vi "RT Game POX.vi"() -> ()   [LabVIEW 2026]
uses:
  RT State.ctl
  SideSelector.ctl
  <extravilib>/ChannelInstances/Tag-bool/Read With Abort.vi
  <extravilib>/ChannelInstances/Tag-bool/Write With Abort.vi
  <vilib>/FPGAPlugInAG/cRIO-9047/niLvFpga_Open_cRIO-9047.vi
  <extravilib>/ChannelInstances/Tag-bool/Instantiate.vi
  <extravilib>/ChannelInstances/Tag-bool/EndpointRead.vi
  <vilib>/Utility/error.llb/Error Cluster From Error Code.vi
  <vilib>/rvi/errors/niLvFpgaAdjustHostInterfaceError.vi
  <extravilib>/ChannelInstances/Tag-bool/Endpoint.vi
  <vilib>/rvi/interface/nirviOpenFPGA/nirviOpenFPGA.xnode
  FPGA Bitfiles/speedofvight_FPGATarget_SpeedofVIightFPG_0-Md8D0SXKo.lvbitx
  VSandbox/Speed of VIight FPGA_v2.vi
  <vilib>/rvi/interface/nirviReadWriteControl/nirviReadWriteControl.xnode
  NiFpgaLv.dll
  <extravilib>/ChannelInstances/Tag-bool.lvlib
panel:
  in  "Effect":T1(ring)
  in  "Complete Game":bool
  in  "Abort Game":bool
  out "Player 2 Score Live":u32
  out "Player 1 Score Live":u32
  out "Player 2 Score":u32
  out "Player 1 Score":u32
  out "Enum":T2=enum."Game<>Conclude"
  in  "Game Length (s)":u32=2
  in  "Bonus Threshold":u64=30000
  in  "Commit to Game":bool
  in  "Stop Idle":bool
  out "Closing Loop":i32
  out "Main Loop":i32
  out "Idle Loop":i32
  in  "stop":bool
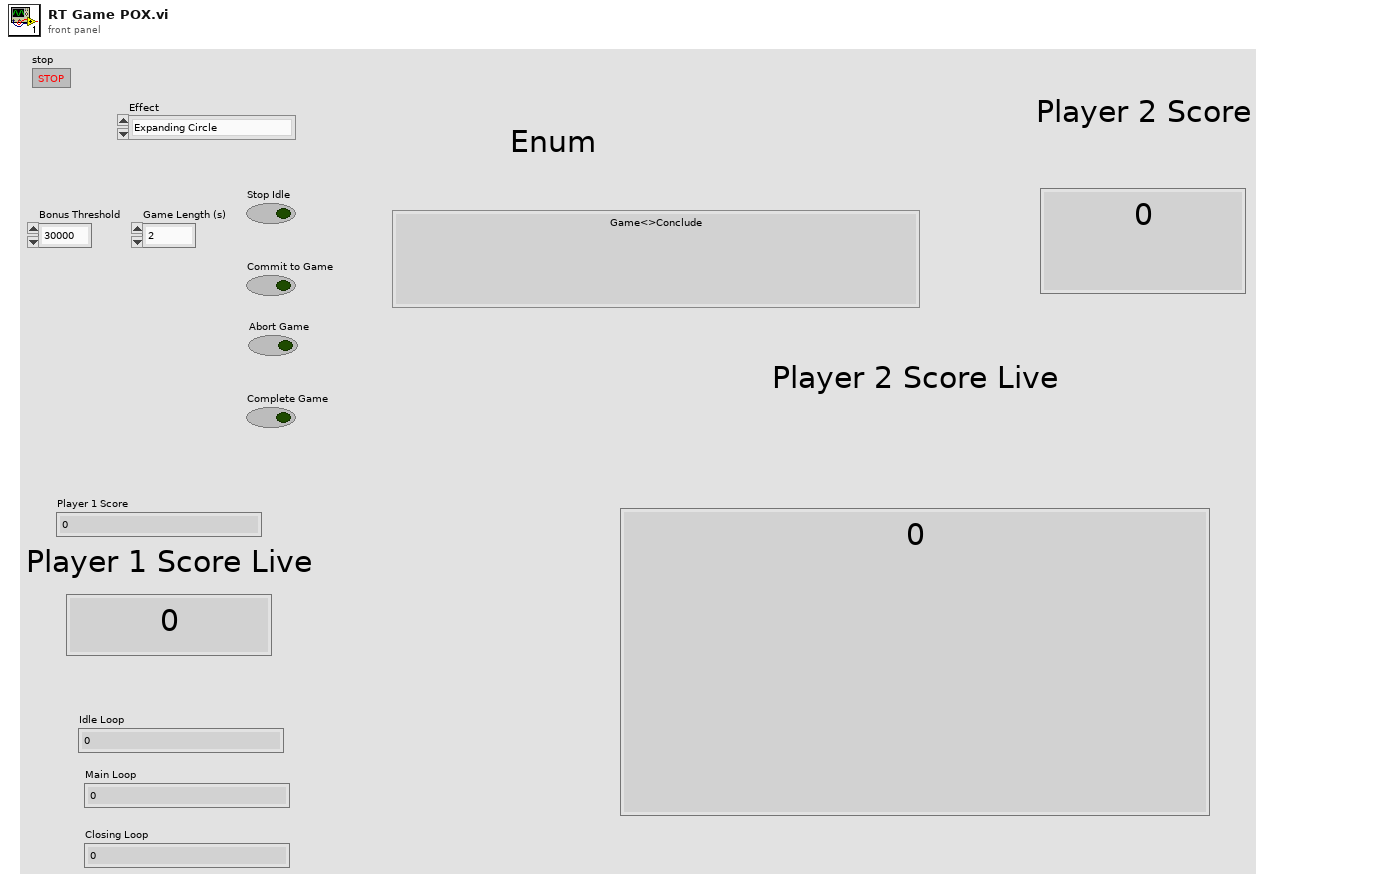
[diagram p1: front panel]
types:
  T1 = enum16{"Expanding Circle", "Plasma", "Radar Sweep", "Matrix Rain", "Campfire", "Diagonal Scan"}
  T2 = typedef "RT State.ctl" = enum16{"<Startup>", "Idle", "Configuring", "Game<>Countdown", "Game<>Play", "Game<>Conclude"}
  T3 = typedef "SideSelector.ctl" = enum16{"P12", "P1", "P2"}
  T4 = typedef "Tag-bool.lvlib/))Channel.ctl" = refnum<queue>
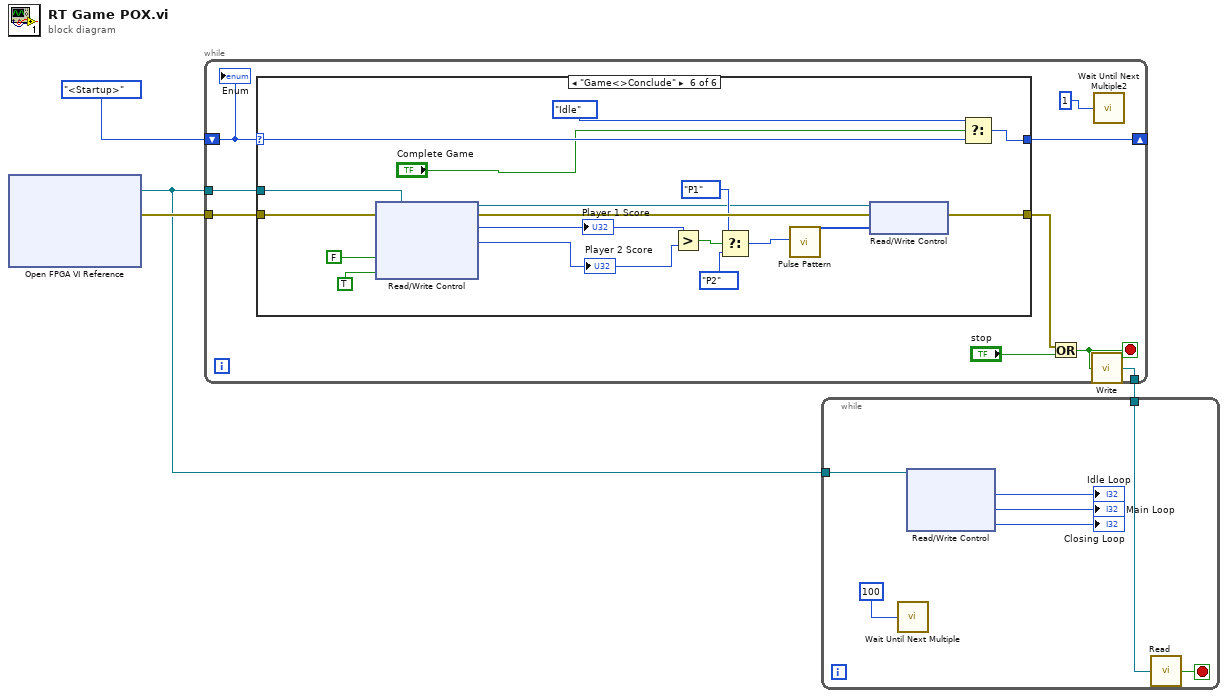
[diagram p0: block diagram]
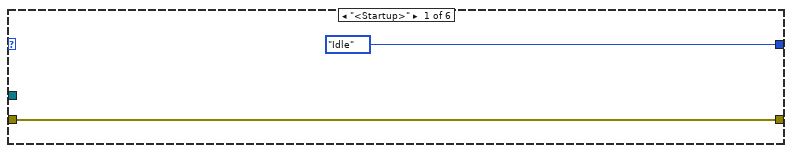
[diagram p2: hidden frame]
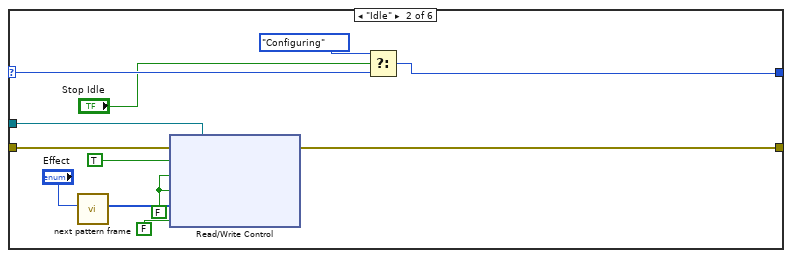
[diagram p3: hidden frame]
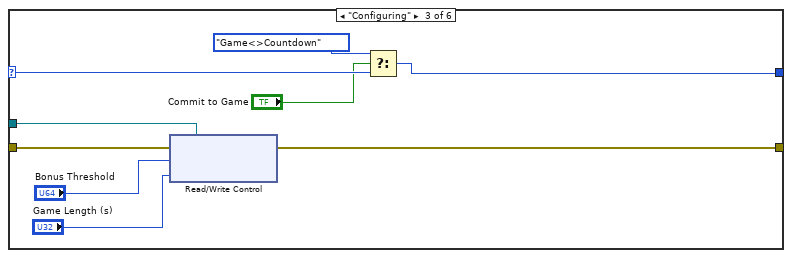
[diagram p4: hidden frame]
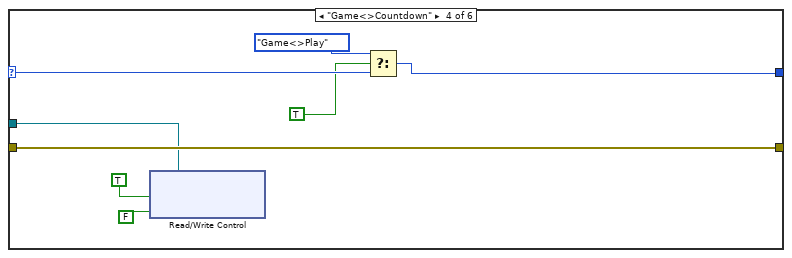
[diagram p5: hidden frame]
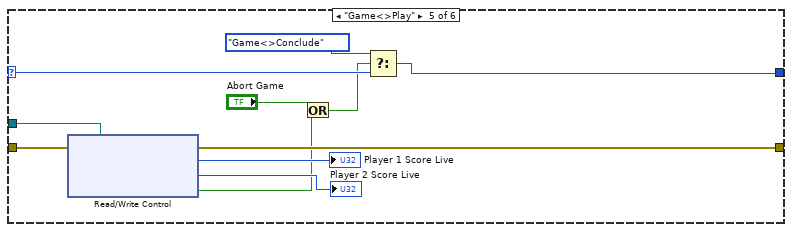
[diagram p6: hidden frame]
diagram:
  n1 = xnode "Open FPGA VI Reference"() -> ("FPGA VI Reference Out"=w2:refnum<k20>, "error out"=w4:errorcluster)  [unwired: 2 in]
  n2 = while {
    tunnel: w4 -> [w13]
    tunnel: w2 -> [w12]
    shift-right: [w9] -> _
    shift-left: RT_State."<Startup>" -> [w6]
    tunnel: [w10] -> w1
    stop <- w8 stop-if-true
    n3 = case shown="\"Game<>Conclude\"" w6 {
      selector: w6 -> [_ w25 w34 w43 w55 w72]
      tunnel: w13 -> [w14 w27 w36 w44 w50 w69]
      tunnel: w12 -> [_ w26 w35 w39 w48 w68]
      tunnel: [RT_State."Idle" w24 w33 w42 w54 w71] -> w9
      tunnel: [w14 w21 w30 w44 w49 w67] -> w7
      frame "<Startup>" {
      }
      frame "Idle" {
        w20 = FALSE ("Stop Idle")
        n4 = call "next pattern frame.vi"("Effect"="Effect") -> ("Array"=w18:u16[])  [unwired: 10 in]
        n5 = xnode "Read/Write Control"("FPGA VI Reference In"=w26, "error in"=w27, "Stop Closing Loop"=TRUE, "Stop Idle"=w20, "Stop Main Loop"=w20, "Idle Pattern"=w18, "Main Loop Complete"=FALSE) -> ("error out"=w21:errorcluster)  [unwired: 1 out]
        n6 = Select(t=RT_State."Configuring", s="Stop Idle", f=w25) -> (s? t:f=w24:T2)
      }
      frame "Configuring" {
        n7 = xnode "Read/Write Control"("FPGA VI Reference In"=w35, "error in"=w36, "Bonus Threshold"="Bonus Threshold", "Game Length (s)"="Game Length (s)") -> ("error out"=w30:errorcluster)  [unwired: 1 out]
        n8 = Select(t=RT_State."Game<>Countdown", s="Commit to Game", f=w34) -> (s? t:f=w33:T2)
      }
      frame "Game<>Countdown" {
        n9 = xnode "Read/Write Control"("FPGA VI Reference In"=w39, "Stop Idle"=TRUE, "Stop Closing Loop"=FALSE) -> ()  [unwired: 1 in, 2 out]
        n10 = Select(t=RT_State."Game<>Play", s=TRUE, f=w43) -> (s? t:f=w42:T2)
      }
      frame "Game<>Play" {
        n11 = xnode "Read/Write Control"("FPGA VI Reference In"=w48, "error in"=w50) -> ("error out"=w49:errorcluster, "Player 1 Score"=→"Player 1 Score Live":u32, "Player 2 Score"=→"Player 2 Score Live":u32, "Main Loop Complete"=w45:bool)  [unwired: 1 out]
        n12 = Or(x="Abort Game", y=w45) -> (x .or. y?=w46:bool)
        n13 = Select(t=RT_State."Game<>Conclude", s=w46, f=w55) -> (s? t:f=w54:T2)
      }
      frame "Game<>Conclude" {
        n14 = xnode "Read/Write Control"("FPGA VI Reference In"=w68, "error in"=w69, "Stop Idle"=FALSE, "Stop Main Loop"=TRUE) -> ("FPGA VI Reference Out"=w57:refnum<k20>, "error out"=w67:errorcluster, "Player 1 Score"=w63:u32, "Player 2 Score"=w62:u32)
        "Player 1 Score" <- w63
        "Player 2 Score" <- w62
        n15 = Greater?(x=w63, y=w62) -> (0:w61:bool)
        n16 = Select(t=SideSelector."P1" ("Selector"), s=w61, f=SideSelector."P2" ("Selector")) -> (s? t:f=w58:T3)
        n17 = call "Pulse Pattern.vi"("Selector"=w58) -> ("Array"=w56:u16[])  [unwired: 10 in]
        n18 = xnode "Read/Write Control"("FPGA VI Reference In"=w57, "Idle Pattern"=w56) -> ()  [unwired: 1 in, 2 out]
        n19 = Select(t=RT_State."Idle", s="Complete Game", f=w72) -> (s? t:f=w71:T2)
      }
    }
    n20 = Or(x=w7, y="stop") -> (x .or. y?=w8:bool)
    n21 = call <extravilib>:"Write.vi"("element"=w8) -> ("channel"=w10:T4)  [unwired: 1 out]
    n22 = call "Wait Until Next Multiple2"("Count(mSec)"=u32 1 ("Count(Ticks)")) -> ()  [unwired: 1 out]
    "Enum" <- w6
  }
  n23 = while {
    tunnel: w2 -> [w79]
    tunnel: w1 -> [w78]
    stop <- w77 stop-if-true
    n24 = call "Wait Until Next Multiple"("Count(mSec)"=u32 100 ("Count(Ticks)")) -> ()  [unwired: 1 out]
    n25 = xnode "Read/Write Control"("FPGA VI Reference In"=w79) -> ("Idle Loop"=→"Idle Loop":i32, "Main Loop"=→"Main Loop":i32, "Closing Loop"=→"Closing Loop":i32)  [unwired: 1 in, 2 out]
    n26 = call <extravilib>:"Read.vi"("channel"=w78) -> ("element"=w77:bool)  [unwired: 1 in, 1 out]
  }
